vi "Shutdown.vi"(8 "error in":errorcluster, 11 "cPAS in":refnum<class "cPAS.lvclass">) -> (0 "error out":errorcluster, 3 "cPAS out":refnum<class "cPAS.lvclass">)   [LabVIEW 2015, in "cPAS.lvclass"]
doc: "Shutoff the DC power which will control all outputs, close all references to DAQmx tasks and shutoff the laser AO."
uses:
  cPAS.lvclass
  Reusable/Session Log/System Log.lvclass
  Reusable/Session APIs/File Access/Config Data/Config Data.lvclass
  Reusable/Instrument/Instrument.lvclass/Instrument.ctl
  Reusable/Instrument/Read Log Session.vi
  Reusable/Instrument/Read Cfg Session.vi
  Read Serial IO.vi
  Read tecEn.vi
  Read tecSP.vi
  Read FPGA_Ref.vi
  <vilib>/Utility/error.llb/Error Cluster From Error Code.vi
  <vilib>/rvi/errors/niLvFpgaAdjustHostInterfaceError.vi
  Reusable/PAS/Main/PAS.lvclass
  Devices/Configurable Device/Configurable Device.lvclass
  Interface/fpga_ctl.ctl
  <userlib>/_Session Fwk/Session - Root.lvclass
  <vilib>/rvi/interface/nirviMethod/nirviMethod.xnode
  FPGA Bitfiles/FPGA Server.lvbitx
  <vilib>/rvi/interface/nirviReadWriteControl/nirviReadWriteControl.xnode
  <vilib>/FPGAPlugInAG/PXI-7841R/niLvFpga_StopFifo_PXI-7841R.vi
  <vilib>/rvi/errors/niLvFpgaMergeErrorWithErrorCode.vi
  NiFpgaLv.dll
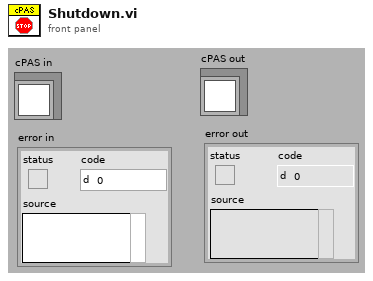
[diagram p1: front panel]
types:
  T1 = typedef "fpga_ctl.ctl" = refnum<k20>
  T2 = typedef "Session - Root.lvclass/Session Handle.ctl" = refnum<data-value>
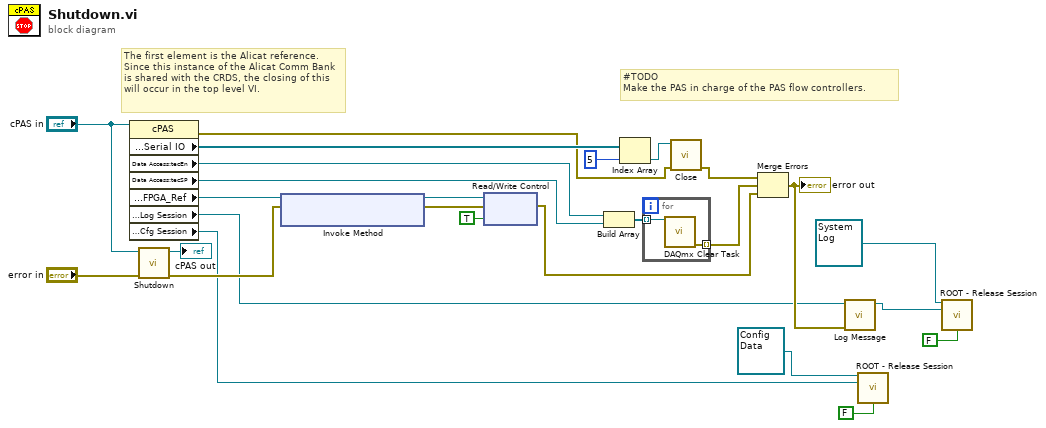
[diagram p0: block diagram]
diagram:
  # "#TODO\nMake the PAS in charge of the PAS flow controllers."
  # "The first element is the Alicat reference.  Since this instance of the Alicat Comm Bank is shared with the CRDS, the closing of this will occur in the top level VI."
  n1 = property class="cPAS"(reference="cPAS in") -> (error out=w10:errorcluster, "Data Access:Serial IO"=w13:refnum<class "Configurable Device.lvclass">[], "Data Access:tecEn"=w25:refnum<k21>, "Data Access:tecSP"=w24:refnum<k21>, "Data Access:FPGA_Ref"=w19:T1, "Accessors:Log Session"=w7:T2, "Accessors:Cfg Session"=w2:T2)  [unwired: 1 in, 1 out]
  n2 = call-parent "Shutdown.vi"("error in"="error in", "Instrument in"="cPAS in") -> ("error out"=w15:errorcluster, "Instrument out"=→"cPAS out":refnum<class "cPAS.lvclass">)  [unwired: 8 in]
  n3 = xnode "Invoke Method"("FPGA VI Reference In"=w19, "error in"=w15) -> ("FPGA VI Reference Out"=w18:T1, "error out"=w17:errorcluster)
  n4 = xnode "Read/Write Control"("FPGA VI Reference In"=w18, "error in"=w17, "stop"=TRUE) -> ("error out"=w14:errorcluster)  [unwired: 1 out]
  n5 = Build Array(w25, w24) -> (w23:refnum<k21>[])
  n6 = Index Array(array=w13, index=5) -> (element=w11:refnum<class "Configurable Device.lvclass">)
  n7 = for {
    tunnel: w23 -> [w28] mode=indexing
    tunnel: [w27] -> w22 mode=indexing
    n8 = call <vilib>:"DAQmx Clear Task.vi"("task in"=w28) -> ("error out"=w27:errorcluster)  [unwired: 14 in]
  }
  n9 = call-dynamic "Close.vi"("error in"=w10, "Cfg Dev in"=w11) -> ("error out"=w9:errorcluster)  [unwired: 8 in, 1 out]
  n10 = Merge Errors(w9, w22, w14) -> (w8:errorcluster)
  "error out" <- w8
  n11 = call "Log Message.vi"("error in"=w8, "session in"=w7) -> ("session out"=w6:T2)  [unwired: 8 in, 1 out]
  n12 = call <userlib>:"ROOT - Release Session.vi"("OBJ - Session in"=refnum<class "Config Data.lvclass"> refnum ("Config Data"), "Session Handle in"=w2, "force destroy? (F)"=FALSE) -> ()  [unwired: 11 in, 2 out]
  n13 = call <userlib>:"ROOT - Release Session.vi"("OBJ - Session in"=refnum<class "System Log.lvclass"> refnum ("Sys Log"), "Session Handle in"=w6, "force destroy? (F)"=FALSE) -> ()  [unwired: 11 in, 2 out]
